vi "Shutter operate.vi"(0 "Shutters":T1[](array[typedef]), 2 "Open?":bool, 5 "error in":errorcluster) -> (8 "error out":errorcluster)   [LabVIEW 2011]
doc: "Opens or closes one or more shutters connected to a digital I/O board.\n\nThe names of the shutters and the ports to which they are connected to are hard-coded into this vi."
uses:
  new-h-nu-ixon/Laser type.ctt
  <vilib>/DAQmx/write.llb/DAQmx Write (Digital Bool 1Line 1Point).vi
  newhnu shutters/hardware status globals.vi
  <vilib>/DAQmx/create/channels.llb/DAQmx Create Channel (DO-Digital Output).vi
  <vilib>/DAQmx/miscellaneous.llb/DAQmx Fill In Error Info.vi
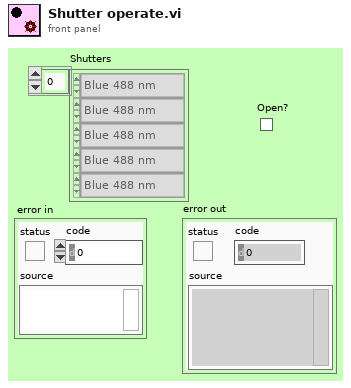
[diagram p1: front panel]
types:
  T1 = typedef "Laser type.ctt" = enum16{"Blue 488 nm", "Green 532 nm", "Red 633 nm", "IR 780"}
  T2 = typedef "shutters status.ctl" = cluster{"Laser":T1, "Status":bool}[]
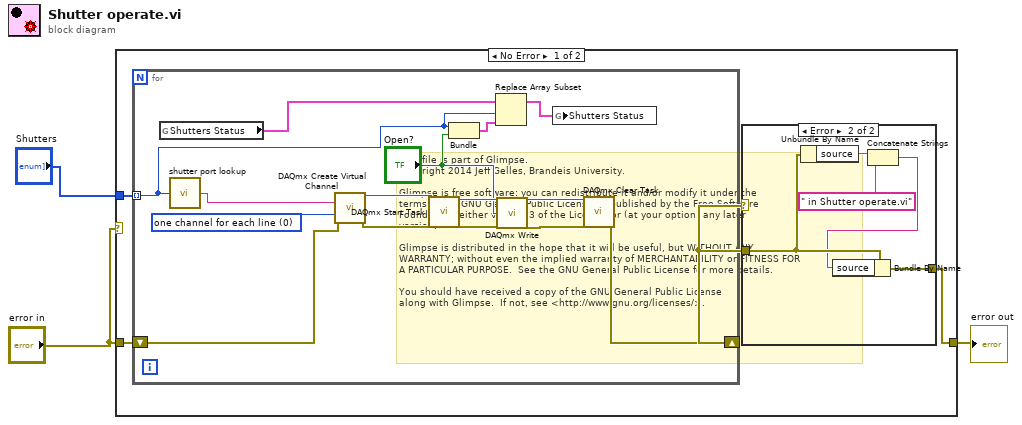
[diagram p0: block diagram]
diagram:
  # "This file is part of Glimpse. \nCopyright 2014 Jeff Gelles, Brandeis University.    \n\nGlimpse is free software: you can redistribute it and/or modify it under the \nterms of the GNU General Public License as published by the Free Software \nFoundation, either version 3 of the License, or (at your option) any later \nversion.\n\nGlimpse is distributed in the hope that it will be useful, but WITHOUT ANY \nWARRANTY; without even the implied warranty of MERCHANTABILITY or FITNESS FOR \nA PARTICULAR PURPOSE.  See the GNU General Public License for more details.\n\nYou should have received a copy of the GNU General Public License\nalong with Glimpse.  If not, see <http://www.gnu.org/licenses/>."
  n1 = case shown="No Error" "error in" {
    tunnel: "error in" -> [w7 w29]
    tunnel: [w5 w29] -> w3
    tunnel: "Shutters" -> [w6 _]
    frame No Error {
      n2 = for {
        tunnel: w6 -> [w15] mode=indexing
        shift-right: [w19] -> w4
        shift-left: w7 -> [w20]
        w22 = 0 items=["one channel for each line", "one channel for all lines"] ("line grouping")
        n3 = global read "hardware status globals.vi" "Shutters Status"() -> (w17:T2)
        n4 = call "shutter port lookup.vi"("Shutter name"=w15) -> ("Shutter Device and port"=w21:tag)
        n5 = call-poly <vilib>:"DAQmx Create Virtual Channel.vi"("lines"=w21, "line grouping"=w22, "error in"=w20) -> ("task out"=w24:refnum<k21>, "error out"=w23:errorcluster)  [unwired: 4 in, 7 out]
        n6 = call <vilib>:"DAQmx Start Task.vi"("task/channels in"=w24, "error in"=w23) -> ("task out"=w26:refnum<k21>, "error out"=w28:errorcluster)  [unwired: 12 out]
        n7 = Bundle("Enum"=w15, "Open?") -> (w16:cluster{"Enum":T1, bool})  [unwired: 1 out]
        n8 = Replace Array Subset(array=w17, new element=w16, index=w15) -> (w14:T2)
        n9 = call-poly <vilib>:"DAQmx Write.vi"("task/channels in"=w26, "data"="Open?", "error in"=w28) -> ("task out"=w25:refnum<k21>, "error out"=w27:errorcluster)  [unwired: 1 in, 10 out]
        n10 = global write "hardware status globals.vi" "Shutters Status"(w14) -> ()
        n11 = call <vilib>:"DAQmx Clear Task.vi"("task in"=w25, "error in"=w27) -> ("error out"=w19:errorcluster)  [unwired: 13 out]
      }
      n12 = case shown="Error" w4 {
        tunnel: w4 -> [w8 w12]
        tunnel: [w8 w13] -> w5
        frame No Error {
        }
        frame Error {
          n13 = Unbundle By Name(w12) -> ("source"=w11:string)
          n14 = Concatenate Strings(w11, " in Shutter operate.vi" ("string")) -> (w9:string)
          n15 = Bundle By Name(cluster=w12, "source"=w9) -> (w13:errorcluster)
        }
      }
    }
    frame Error {
    }
  }
  "error out" <- w3
